vi "Execute.vi"(8 "error in":errorcluster, 9 "Consumer Queues in":T1, 10 "DAC Process Command in":refnum<class "Run DAC Front Panel.lvclass">, 11 "DAC Process Data in":T2) -> (0 "error out":errorcluster, 1 "Consumer Queues out":T1, 2 "Stop?":bool, 3 "DAC Process Data out":T2)   [LabVIEW 2019, in "DAC Process.lvlib" / "Run DAC Front Panel.lvclass"]
uses:
  Run DAC Front Panel.lvclass
  DAC Process Data.ctl
  Generic Test Stand/Generic Test Stand.lvclass
  TS Framework/ExeLogging/DAC Logger/DAC Logger.lvclass
  DAC State.ctl
  TS Framework/Consumer Queues.ctl
  UI Process/Generic UI Command/Generic UI Process Command.lvclass
  Generic DAC Command/Generic DAC Process Command.lvclass
  Trig Process/Generic Trig Command/Generic Trig Process Command.lvclass
  UI Process/UI Display TS Panel/UI Display TS Panel.lvclass
  Run DAC Front Panel.lvclass/Run DAC Front Panel.ctl
  Generic Test Stand/Generic Test Stand.lvclass/Generic Test Stand.ctl
  UI Process/UI Display TS Panel/UI Display TS Panel.lvclass/UI Display TS Panel.ctl
  Configure DAC Test Stand/Configure DAC Test Stand.lvclass
  DAC Process.lvlib
  TS Framework/TS Framework.lvlib
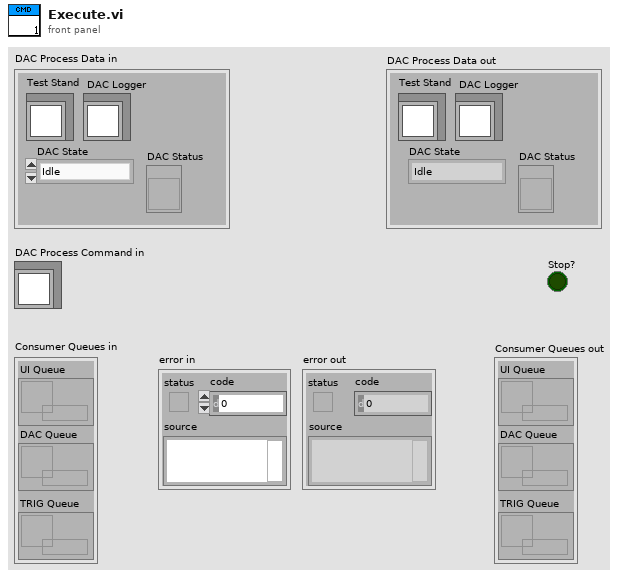
[diagram p1: front panel]
types:
  T1 = typedef "TS Framework.lvlib/Consumer Queues.ctl" = cluster{"UI Queue":refnum<queue>, "DAC Queue":refnum<queue>, "TRIG Queue":refnum<queue>}
  T2 = typedef "DAC Process.lvlib/DAC Process Data.ctl" = cluster{"Test Stand":refnum<class "Generic Test Stand.lvclass">, " DAC Logger":refnum<class "DAC Logger.lvclass">, "DAC State":T3, "DAC Status":refnum<vi>}
  T3 = typedef "DAC Process.lvlib/DAC State.ctl" = enum16{"Idle", "Acquiring"}
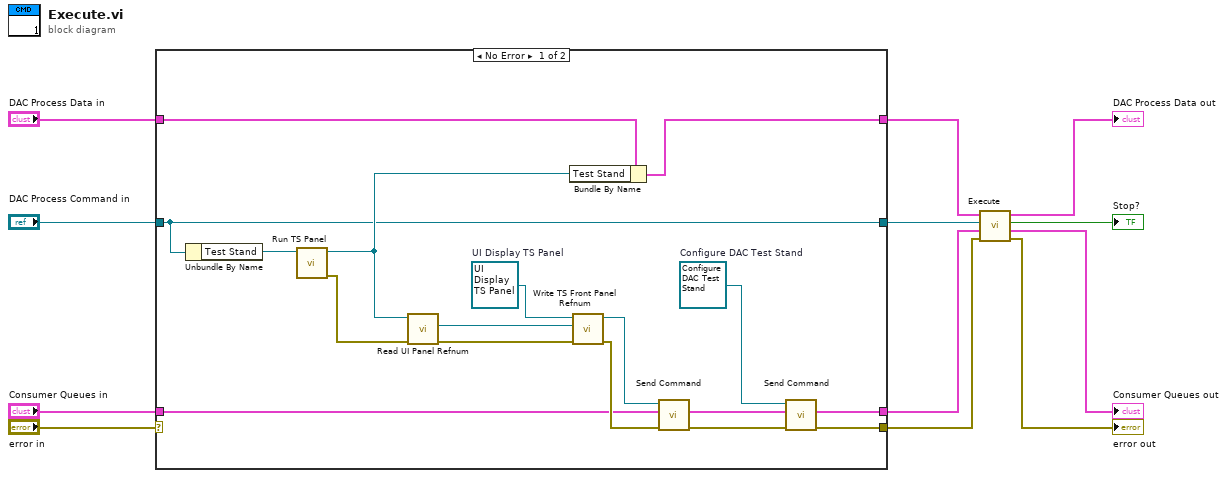
[diagram p0: block diagram]
diagram:
  n1 = case shown="No Error" "error in" {
    selector: "error in" -> [_ w31]
    tunnel: "DAC Process Command in" -> [w18 w30]
    tunnel: "DAC Process Data in" -> [w25 w33]
    tunnel: [w24 w33] -> w5
    tunnel: "Consumer Queues in" -> [w19 w32]
    tunnel: [w15 w32] -> w3
    tunnel: [w14 w31] -> w2
    tunnel: [w18 w30] -> w1
    frame No Error {
      w13 = refnum<class "Configure DAC Test Stand.lvclass"> refnum  # Configure DAC Test Stand
      w29 = refnum<class "UI Display TS Panel.lvclass"> refnum  # UI Display TS Panel
      n2 = Unbundle By Name(w18) -> ("Test Stand"=w26:refnum<class "Generic Test Stand.lvclass">)
      n3 = call-dynamic "Run TS Panel.vi"("Generic Test Stand in"=w26) -> ("error out"=w22:errorcluster, "Generic Test Stand out"=w23:refnum<class "Generic Test Stand.lvclass">)  [unwired: 9 in]
      n4 = call "Read UI Panel Refnum.vi"("error in (no error)"=w22, "Generic Test Stand in"=w23) -> ("error out"=w21:errorcluster, "UI Panel Refnum"=w27:refnum<vi>)  [unwired: 7 in, 1 out]
      n5 = Bundle By Name(cluster=w25, "Test Stand"=w23) -> (w24:T2)
      n6 = call "Write TS Front Panel Refnum.vi"("error in (no error)"=w21, "TS Front Panel Refnum"=w27, "UI Display TS Panel in"=w29) -> ("error out"=w20:errorcluster, "UI Display TS Panel out"=w28:refnum<class "UI Display TS Panel.lvclass">)  [unwired: 7 in]
      n7 = call-dynamic "Send Command.vi"("error in (no error)"=w20, "Consumer Queues in"=w19, "UI Process Command in"=w28) -> ("error out"=w16:errorcluster, "Consumer Queues out"=w17:T1)  [unwired: 7 in]
      n8 = call-dynamic "Send Command.vi"("error in (no error)"=w16, "Consumer Queues in"=w17, "DAC Process Command"=w13) -> ("error out"=w14:errorcluster, "Consumer Queues out"=w15:T1)  [unwired: 7 in]
    }
    frame Error {
    }
  }
  n9 = call-parent "Execute.vi"("error in"=w2, "Consumer Queues in"=w3, "DAC Process Command in"=w1, "DAC Process Data in"=w5) -> ("error out"=→"error out":errorcluster, "Consumer Queues out"=→"Consumer Queues out":T1, "Stop?"=→"Stop?":bool, "DAC Process Data out"=→"DAC Process Data out":T2)  [unwired: 4 in]
